vi "Convert time.vi"(10 "date time rec":T1) -> (2 "date time rec 2":T1)   [LabVIEW 2020]
uses:
  <vilib>/Utility/miscctls.llb/LVDateTimeRec.ctl
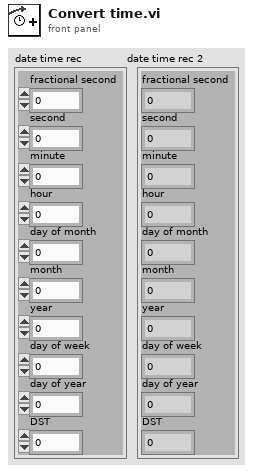
[diagram p1: front panel]
types:
  T1 = typedef "LVDateTimeRec.ctl" = cluster{"fractional second":dbl, "second":i32, "minute":i32, "hour":i32, "day of month":i32, "month":i32, "year":i32, "day of week":i32, "day of year":i32, "DST":i32}
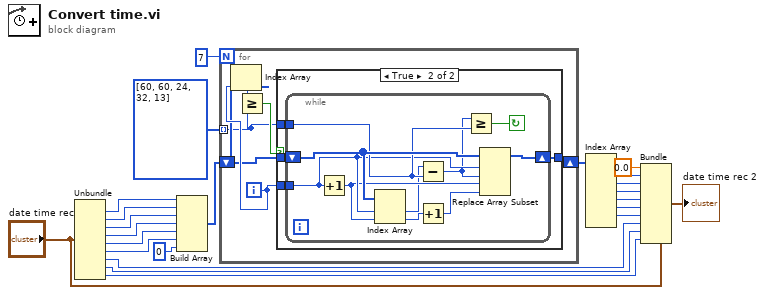
[diagram p0: block diagram]
diagram:
  n1 = Unbundle("date time rec") -> ("second"=w23:i32, "minute"=w22:i32, "hour"=w21:i32, "day of month"=w20:i32, "month"=w19:i32, "year"=w18:i32, "day of week"=w6:i32, "day of year"=w5:i32, "DST"=w4:i32)  [unwired: 1 out]
  n2 = Build Array(w23, w22, w21, w20, w19, w18, 0 ("element")) -> (w16:i32[])
  n3 = for {
    N: 7 -> [_]
    tunnel: i32[] [60, 60, 24, 32, 13] -> [w24] mode=indexing
    shift-right: [w29] -> w13
    shift-left: w16 -> [w26]
    i -> [w27]
    n4 = Index Array(array=w26, index=w27) -> (element=w25:i32)
    n5 = Greater Or Equal?(x=w25, y=w24) -> (x >= y?=w28:bool)
    n6 = case shown="True" w28 {
      tunnel: w24 -> [_ w34]
      tunnel: w27 -> [_ w33]
      tunnel: w26 -> [w30 w32]
      tunnel: [w30 w31] -> w29
      frame False {
      }
      frame True {
        n7 = while {
          tunnel: w34 -> [w41]
          tunnel: w33 -> [w40]
          shift-right: [w43] -> w31
          shift-left: w32 -> [w42]
          stop <- w44 continue-if-true
          n8 = Increment(x=w40) -> (x+1=w39:i32)
          n9 = Index Array(array=w42, index #1=w40, index #2=w39) -> (element #1=w36:i32, element #2=w38:i32)
          n10 = Subtract(x=w36, y=w41) -> (x-y=w35:i32)
          n11 = Increment(x=w38) -> (x+1=w37:i32)
          n12 = Greater Or Equal?(x=w35, y=w41) -> (x >= y?=w44:bool)
          n13 = Replace Array Subset(array=w42, new element #1=w35, index #1=w40, new element #2=w37, index #2=w39) -> (w43:i32[])
        }
      }
    }
  }
  n14 = Index Array(array=w13) -> (element #1=w12:i32, element #2=w11:i32, element #3=w10:i32, element #4=w9:i32, element #5=w8:i32, element #6=w7:i32)  [unwired: 7 in, 1 out]
  n15 = Bundle(cluster="date time rec", "fractional second"=0.0, "second"=w12, "minute"=w11, "hour"=w10, "day of month"=w9, "month"=w8, "year"=w7, "day of week"=w6, "day of year"=w5, "DST"=w4) -> (→"date time rec 2":T1)
